vi "Get monitor scale.vi"(11 "Monitor scale":dbl=43.0) -> (2 "OK":bool, 3 "Monitor scale out":dbl)   [LabVIEW 2012]
panel:
  in  "Cancel":bool
  in  "OK":bool
  in  "Monitor scale edit":dbl=43.0 caption="Monitor scale:"
  out "Bars":picture
  # "Adjust the monitor scale until the bars are 2cm wide."
  # "pix/cm"
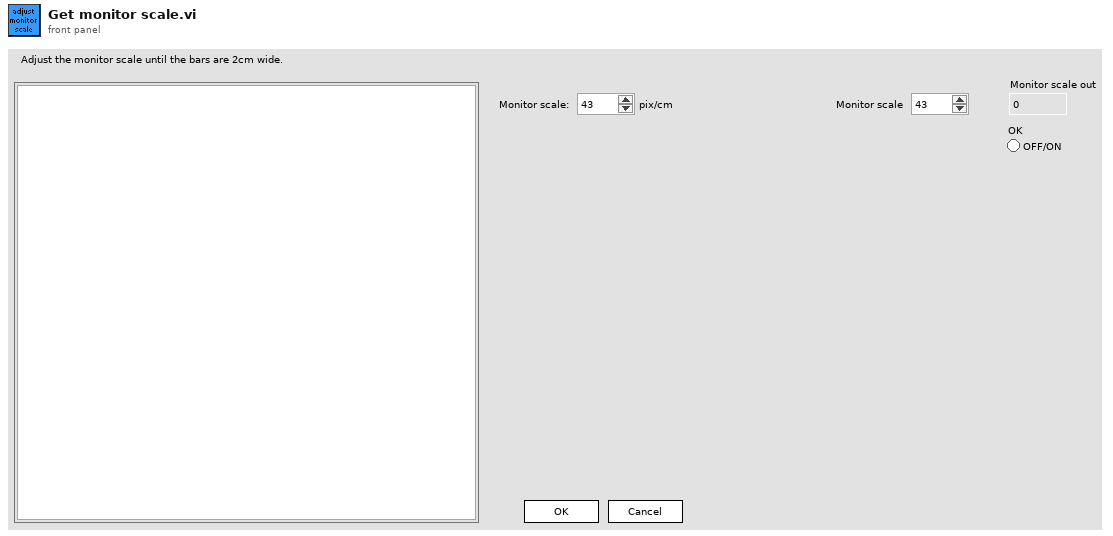
[diagram p1: front panel]
types:
  T1 = typedef "LVBoundsTypeDef.ctl" = cluster{"Width":u32, "Height":u32}
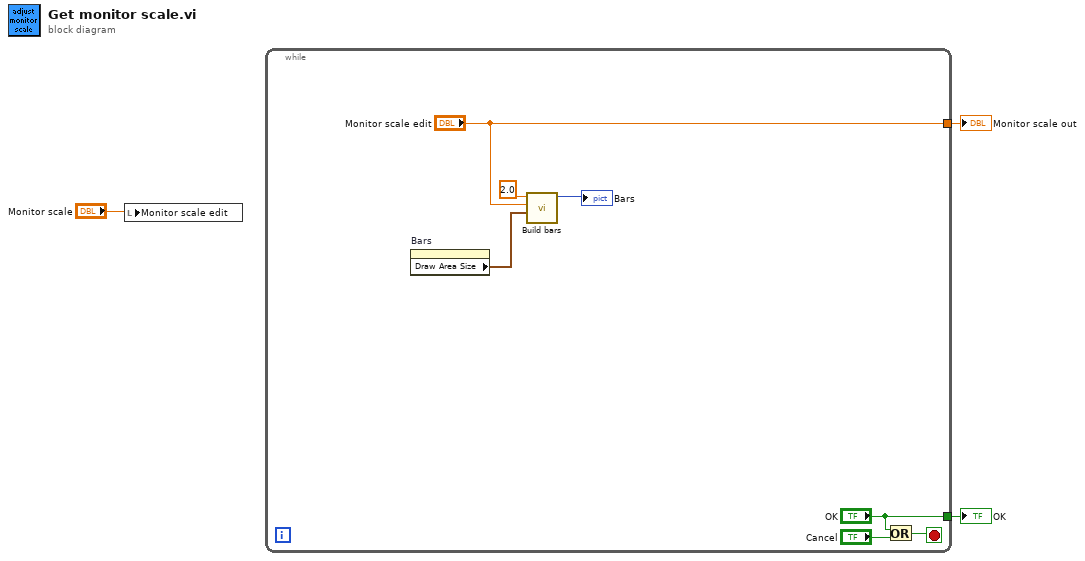
[diagram p0: block diagram]
diagram:
  n1 = local write "Monitor scale edit"("Monitor scale") -> ()
  n2 = while {
    tunnel: ["OK"] -> w2
    tunnel: ["Monitor scale edit"] -> w3
    stop <- w10 stop-if-true
    n3 = property on="Bars" class="Pict"() -> ("Draw Area Size"=w7:T1)  [unwired: 2 in, 2 out]
    n4 = call "Build bars.vi"("Draw Area Size"=w7, "Monitor scale"="Monitor scale edit", "Bar width"=2.0) -> ("bars"=→"Bars":picture)  [unwired: 8 in]
    n5 = Or(x="OK", y="Cancel") -> (x .or. y?=w10:bool)
  }
  "Monitor scale out" <- w3
  "OK" <- w2
